vi "Receive Message.vi"(6 "timeout in ms (-1)":i32=-1, 8 "error in":errorcluster, 11 "IMessageTransport in":refnum<class "IMessageTransport.lvclass">) -> (0 "error out":errorcluster, 2 "Q Element":refnum<class "IMessagePayload.lvclass">, 3 "IMessageTransport out":refnum<class "IMessageTransport.lvclass">)   [LabVIEW 2016, in "IMessageTransport.lvclass"]
uses:
  IMessageTransport.lvclass
  IMessagePayload/IMessagePayload.lvclass
  QMHMessagePayload/QMHMessagePayload.lvclass
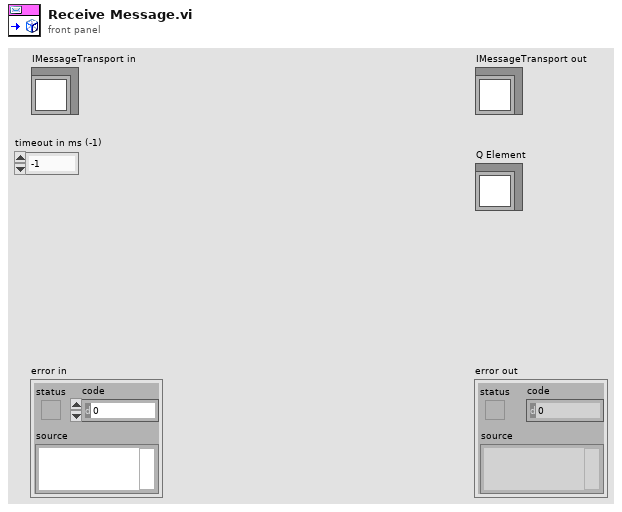
[diagram p1: front panel]
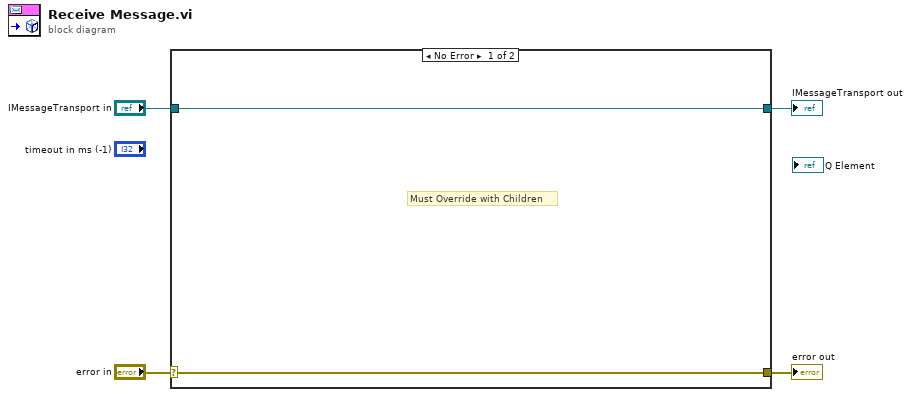
[diagram p0: block diagram]
diagram:
  n1 = case shown="No Error" "error in" {
    selector: "error in" -> [w5 w8]
    tunnel: [w5 w8] -> w3
    tunnel: [w6 w7] -> w1
    tunnel: "IMessageTransport in" -> [w6 w7]
    frame No Error {
      # "Must Override with Children"
    }
    frame Error {
    }
  }
  "error out" <- w3
  "IMessageTransport out" <- w1
